vi "PostObjectTerminate.vi"(8 "error in (no error)":errorcluster, 11 "AFM_Driver in":refnum<class "AFM_Driver.lvclass">) -> (0 "error out":errorcluster, 3 "AFM_Driver out":refnum<class "AFM_Driver.lvclass">)   [LabVIEW 2019, in "AFM_Driver.lvclass"]
uses:
  AFM_Driver.lvclass
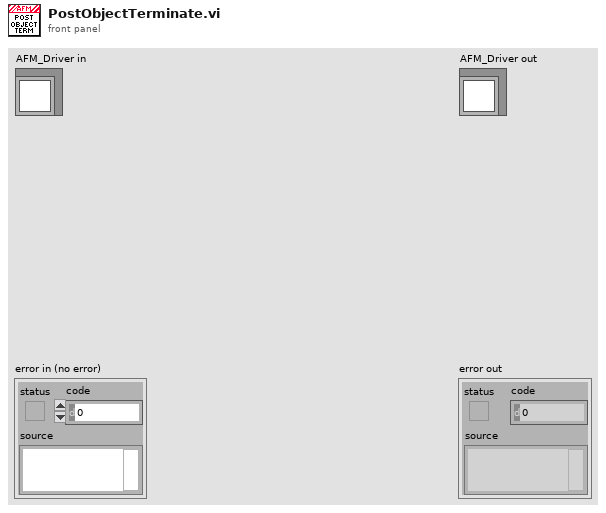
[diagram p1: front panel]
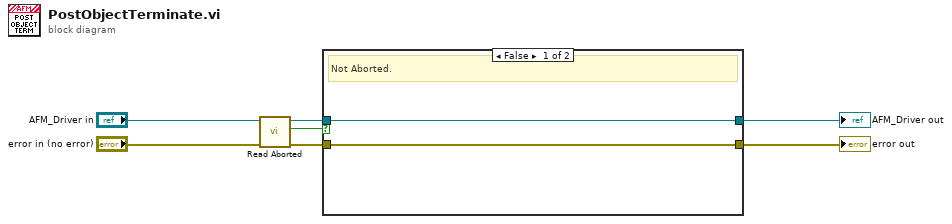
[diagram p0: block diagram]
diagram:
  n1 = call "Read Aborted"("error in (no error)"="error in (no error)", "AFM_Driver in"="AFM_Driver in") -> ("error out"=w5:errorcluster, "Aborted?"=w7:bool, "AFM_Driver out"=w6:refnum<class "AFM_Driver.lvclass">)  [unwired: 7 in]
  n2 = case shown="False" w7 {
    tunnel: w6 -> [w8 w11]
    tunnel: [w8 w11] -> w2
    tunnel: [w9 w10] -> w1
    tunnel: w5 -> [w9 w10]
    frame False {
      # "Not Aborted."
    }
    frame True {
      # "Aborted. This state must stay empty."
    }
  }
  "error out" <- w1
  "AFM_Driver out" <- w2
